vi "Untitled 1.vi"() -> ()   [LabVIEW 2022 SP3]
panel:
  out "x .and. y?":bool
  out "String":string
  out "x = y?":bool
  in  "Aktualna godzina":string="This is a text.\nHere is a new line.\n\nAnd that's another."
  out "Godziny_jako_array":string[](array[string])
  in  "Godziny_otwarcia":string="This is a text.\nHere is a new line.\n\nAnd that's another."
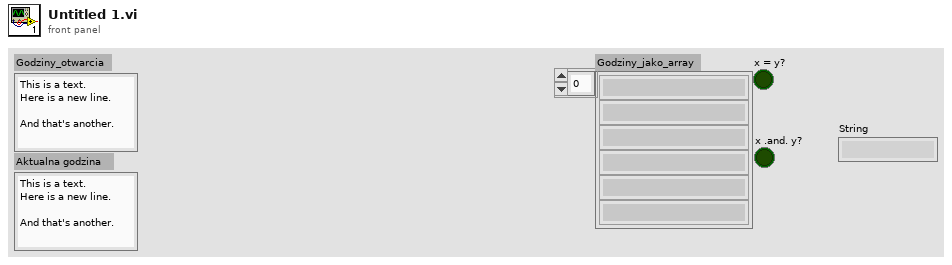
[diagram p1: front panel]
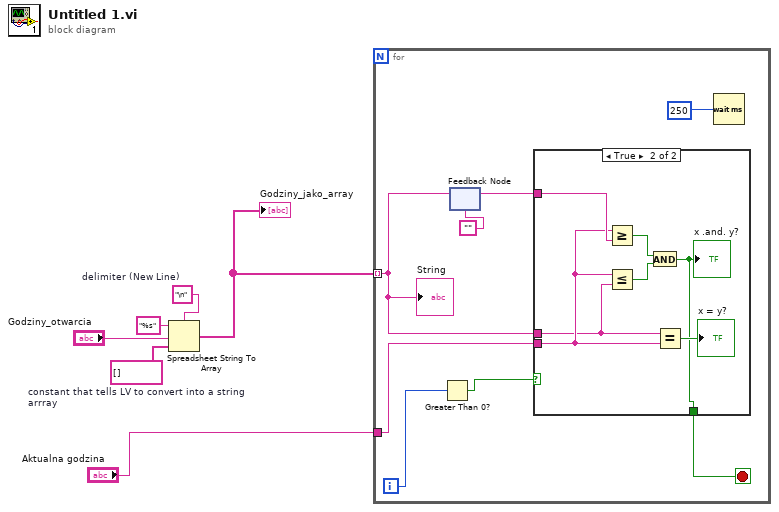
[diagram p0: block diagram]
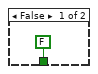
[diagram p2: hidden frame]
diagram:
  w5 = "\n"  # delimiter (New Line)
  w4 = string[] []  # constant that tells LV to convert into a string arrray
  n1 = Spreadsheet String To Array(delimiter (Tab)=w5, format string="%s", spreadsheet string="Godziny_otwarcia", array type (2D Dbl)=w4) -> (array=w2:string[])
  "Godziny_jako_array" <- w2
  n2 = for {
    tunnel: w2 -> [w9] mode=indexing
    tunnel: "Aktualna godzina" -> [w14]
    i -> [w10]
    stop <- w13 stop-if-true
    n3 = Greater Than 0?(x=w10) -> (x > 0?=w11:bool)
    n4 = feedback-in #1(w9) -> ()
    n5 = feedback #1("") -> (w7:string)
    n6 = case shown="True" w11 {
      tunnel: w9 -> [_ w19]
      tunnel: w14 -> [_ w20]
      tunnel: [FALSE w16] -> w13
      tunnel: w7 -> [_ w21]
      frame False {
      }
      frame True {
        n7 = Greater Or Equal?(x=w20, y=w21) -> (x >= y?=w17:bool)
        n8 = Less Or Equal?(x=w20, y=w19) -> (x <= y?=w18:bool)
        n9 = And(x=w17, y=w18) -> (x .and. y?=w16:bool)
        "x .and. y?" <- w16
        n10 = Equal?(x=w19, y=w20) -> (x = y?=→"x = y?":bool)
      }
    }
    n11 = Wait (ms)(milliseconds to wait=u32 250 ("millisecond timer value")) -> ()  [unwired: 1 out]
    "String" <- w9
  }
